vi "MESLog_Result.vi"(0 "ResultID":string, 1 "Barcode":string, 2 "BeginDate":string, 3 "TestPeriod":string, 4 "EndDate":string, 5 "UserID":string, 6 "TotalResult":string, 7 "TfpID":string, 8 "EquipID":string, 9 "CreateDate":string, 10 "ManufactureCode":string, 11 "WXPOnum":string) -> (16 "Result":string)   [LabVIEW 2014]
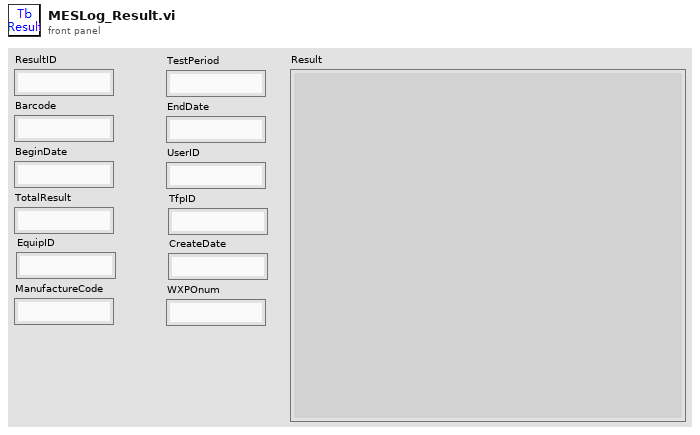
[diagram p1: front panel]
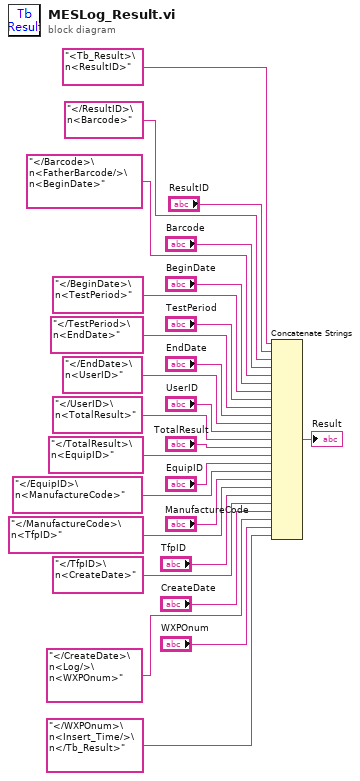
[diagram p0: block diagram]
diagram:
  n1 = Concatenate Strings("<Tb_Result>\n<ResultID>" ("string"), "ResultID", "</ResultID>\n<Barcode>" ("string"), "Barcode", "</Barcode>\n<FatherBarcode/>\n<BeginDate>" ("string"), "BeginDate", "</BeginDate>\n<TestPeriod>" ("string"), "TestPeriod", "</TestPeriod>\n<EndDate>" ("string"), "EndDate", "</EndDate>\n<UserID>" ("string"), "UserID", "</UserID>\n<TotalResult>" ("string"), "TotalResult", "</TotalResult>\n<EquipID>" ("string"), "EquipID", "</EquipID>\n<ManufactureCode>" ("string"), "ManufactureCode", "</ManufactureCode>\n<TfpID>" ("string"), "TfpID", "</TfpID>\n<CreateDate>" ("string"), "CreateDate", "</CreateDate>\n<Log/>\n<WXPOnum>" ("string"), "WXPOnum", "</WXPOnum>\n<Insert_Time/>\n</Tb_Result>" ("string")) -> (→"Result":string)
